vi "Test Process Error Handler Configured.vi"(8 "error in (no error)":errorcluster, 11 "Process Test In":refnum<class "Process Test.lvclass">) -> (0 "error out":errorcluster, 3 "Process Test Out":refnum<class "Process Test.lvclass">)   [LabVIEW 2020, in "Process Test.lvclass"]
uses:
  Process Test.lvclass
  C:/Program Files (x86)/National Instruments/LabVIEW 2020/vi.lib/Asteme/LUnit/Test Case.lvclass
  Mock Error Handler/Mock Error Handler.lvclass
  C:/Users/anton/Documents/GitHub/Triarc-Framework/source/Framework/Error Handler Interface/Error Handler Interface.lvclass
  Framework/Process/Process.lvclass/Process.ctl
  <vilib>/Asteme/LUnit/Test Case.lvclass/Test Case.ctl
  <vilib>/Asteme/LUnit/LUnit Assertion Result.lvclass/LUnit Assertion Result.ctl
  Framework/Process/Protected/Messaging/Enqueue Message.vi
  Framework/Process/Public/Lifecycle/Get Lifecycle State.vi
  <vilib>/Asteme/LUnit/Palette/Fail.vi
  <vilib>/Asteme/LUnit/Palette/Pass.vi
  <vilib>/Asteme/LUnit/Set Assertion Type.vi
  <vilib>/Utility/error.llb/Clear Errors.vi
  <vilib>/Asteme/LUnit/Add test result.vi
  <vilib>/Asteme/LUnit/LUnit Write Passed.vi
  <vilib>/Asteme/LUnit/LUnit Get Test Case.vi
  <vilib>/Asteme/LUnit/Assertion Result/LUnit Get Test Name.vi
  <vilib>/Asteme/LUnit/LUnit Write Message.vi
  <vilib>/Asteme/LUnit/LUnit Write Description.vi
  <vilib>/Asteme/LUnit/LUnit Write Assertion Type.vi
  <vilib>/Asteme/LUnit/Read Test Case Name.vi
  <vilib>/Utility/error.llb/Error Cluster From Error Code.vi
  <vilib>/Asteme/LUnit/LUnit Assertion Result.lvclass
  Framework/Process/Process.lvclass
  <vilib>/Asteme/LUnit/Test Case.lvclass
  C:/Users/anton/Documents/GitHub/Triarc-Framework/source/Framework/Base/Base.lvclass
  C:/Users/anton/Documents/GitHub/Triarc-Framework/source/Framework Test/Mock Error Handler/Mock Error Handler.lvclass
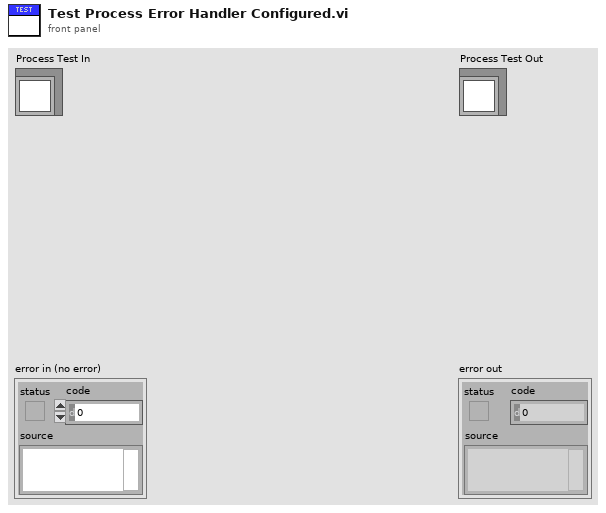
[diagram p1: front panel]
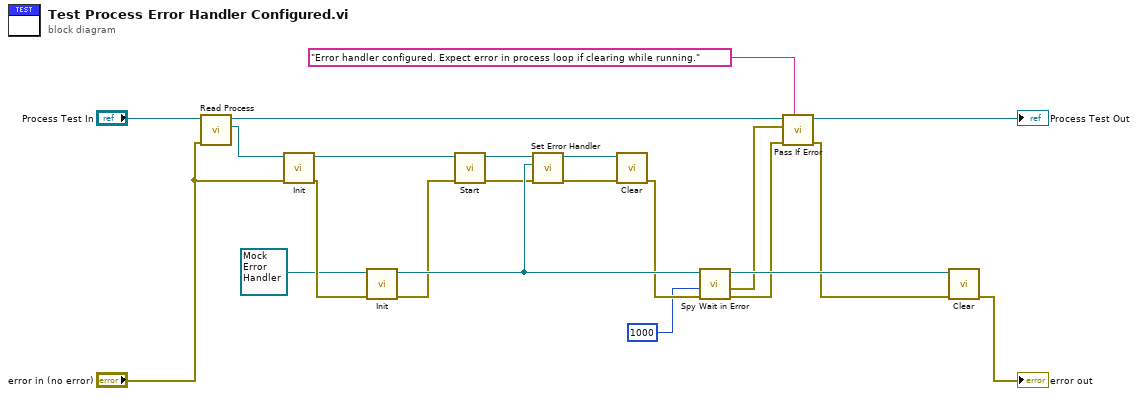
[diagram p0: block diagram]
diagram:
  n1 = call "Read Process.vi"("error in (no error)"="error in (no error)", "Process Test in"="Process Test In") -> ("Process.lvclass"=w9:refnum<class "Process.lvclass">, "Process Test out"=w8:refnum<class "Process Test.lvclass">)  [unwired: 7 in, 1 out]
  n2 = call-dynamic "Init.vi"("error in (no error)"="error in (no error)", "Process In"=w9) -> ("error out"=w21:errorcluster, "Process Out"=w2:refnum<class "Process.lvclass">)  [unwired: 8 in]
  n3 = call-dynamic "Init.vi"("error in (no error)"=w21, "Mock Error Handler In"=refnum<class "Mock Error Handler.lvclass"> refnum ("Mock Error Handler.lvclass")) -> ("error out"=w4:errorcluster, "Mock Error Handler Out"=w17:refnum<class "Mock Error Handler.lvclass">)  [unwired: 8 in]
  n4 = call "Start.vi"("error in (no error)"=w4, "Process In"=w2) -> ("error out"=w3:errorcluster, "Process Out"=w1:refnum<class "Process.lvclass">)  [unwired: 8 in]
  n5 = call "Set Error Handler.vi"("error in (no error)"=w3, "Error Handler"=w17, "Process In"=w1) -> ("error out"=w18:errorcluster, "Process Out"=w19:refnum<class "Process.lvclass">)  [unwired: 7 in]
  n6 = call-dynamic "Clear.vi"("error in (no error)"=w18, "Process In"=w19) -> ("error out"=w14:errorcluster)  [unwired: 9 in]
  n7 = call "Spy Wait in Error.vi"("error in (no error)"=w14, "timeout in ms (-1)"=1000, "Mock Error Handler In"=w17) -> ("error out"=w13:errorcluster, "Errors"=w12:errorcluster, "Mock Error Handler Out"=w16:refnum<class "Mock Error Handler.lvclass">)  [unwired: 4 in, 2 out]
  n8 = call <vilib>:"Pass If Error.vi"("Description"="Error handler configured. Expect error in process loop if clearing while running.", "error in (no error)"=w13, "Assert error"=w12, "Test Case In"=w8) -> ("error out"=w11:errorcluster, "Test Case Out"=→"Process Test Out":refnum<class "Process Test.lvclass">)  [unwired: 6 in]
  n9 = call-dynamic "Clear.vi"("error in (no error)"=w11, "Mock Process In"=w16) -> ("error out"=→"error out":errorcluster)  [unwired: 9 in]
